vi "Find IntelliSense Control [str].vi"(0 "Str Ctl Refnum":refnum<vi>) -> (1 "Found IntelliSenseStringControl":refnum<class "IntelliSenseStringControl.lvclass">, 2 "Other IntelliSense String []":refnum<class "IntelliSenseStringControl.lvclass">[](array[class]), 3 "Found?":bool)   [LabVIEW 2016, in "StringIntelliSense.lvlib" / "IntelliSenseStringControl.lvclass"]
uses:
  IntelliSenseStringControl.lvclass
  IntelliSenseStringControl.lvclass/IntelliSenseStringControl.ctl
  StringMonitorUserData.vi
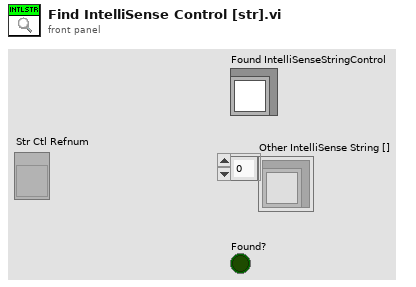
[diagram p1: front panel]
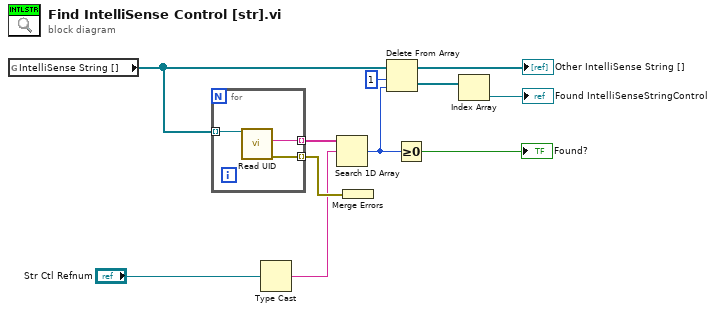
[diagram p0: block diagram]
diagram:
  n1 = global read "StringMonitorUserData.vi" "IntelliSense String []"() -> (w3:refnum<class "IntelliSenseStringControl.lvclass">[])
  n2 = for {
    tunnel: w3 -> [w14] mode=indexing
    tunnel: [w13] -> w11 mode=indexing
    tunnel: [w12] -> w7 mode=indexing
    n3 = call "Read UID.vi"("IntelliSenseStringControl in"=w14) -> ("error out"=w12:errorcluster, "UID"=w13:string)  [unwired: 8 in, 1 out]
  }
  n4 = Type Cast(x="Str Ctl Refnum") -> (*(type *) &x=w1:string)  [unwired: 1 in]
  n5 = Search 1D Array(1D array=w11, element=w1) -> (index of element=w8:i32)  [unwired: 1 in]
  n6 = Merge Errors(w7) -> ()  [unwired: 1 out]
  n7 = Delete From Array(array=w3, length=1, index=w8) -> (deleted portion=w9:refnum<class "IntelliSenseStringControl.lvclass">[], array with subset deleted=→"Other IntelliSense String []":refnum<class "IntelliSenseStringControl.lvclass">[])
  n8 = Greater Or Equal To 0?(x=w8) -> (x >= 0?=→"Found?":bool)
  n9 = Index Array(array=w9) -> (element=→"Found IntelliSenseStringControl":refnum<class "IntelliSenseStringControl.lvclass">)  [unwired: 1 in]
